vi "Bytes to long word.vi"(7 "Index":i32, 9 "Image Data in":u8[](array[numeric])) -> (1 "Index+4":i32, 3 "U32":u32)   [LabVIEW 2014, in "LAVA TIFF File Reader.lvlib"]
uses:
  LAVA TIFF File Reader.lvlib
  Globals.vi
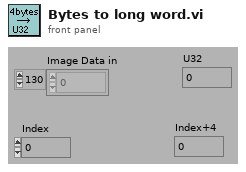
[diagram p1: front panel]
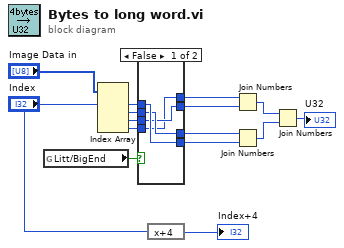
[diagram p0: block diagram]
diagram:
  n1 = global read "Globals.vi" "Litt/BigEnd"() -> (w9:bool)
  n2 = Index Array(array="Image Data in", index #1="Index") -> (element #1=w8:u8, element #2=w6:u8, element #3=w4:u8, element #4=w2:u8)  [unwired: 3 in]
  n3 = case shown="False" w9 {
    tunnel: w8 -> [w19 w20]
    tunnel: [w19 w23] -> w7
    tunnel: w6 -> [w18 w21]
    tunnel: [w18 w22] -> w5
    tunnel: w4 -> [w17 w22]
    tunnel: [w17 w21] -> w3
    tunnel: w2 -> [w16 w23]
    tunnel: [w16 w20] -> w1
    frame False {
    }
    frame True {
    }
  }
  n4 = expression code="x+4"("Index") -> (→"Index+4":i32)
  n5 = Join Numbers(hi=w1, lo=w3) -> ((hi.lo)=w13:u16)
  n6 = Join Numbers(hi=w5, lo=w7) -> ((hi.lo)=w14:u16)
  n7 = Join Numbers(hi=w13, lo=w14) -> ((hi.lo)=→"U32":u32)
